vi "myRIO_BRig_RT__Case_Exp_State_Selection__v4.vi"(0 "input_dataCurrent":u16[](array[numeric]), 1 "input_state":T1, 2 "input_dataExp":u16[](array[numeric]), 5 "input_LickL":bool, 7 "input_FPGA_SelectReward":bool, 9 "input_FPGA_SelectWrong":bool, 11 "input_LickR":bool, 12 "input_arrTrig":bool[](array[boolean])) -> (3 "output_state":T1, 4 "output_dataCurrent":u16[](array[numeric]), 10 "output_LC_Event_l1":bool, 13 "output_LC_Laser_l2":bool, 14 "output_LC_Event_l2":bool, 15 "output_LC_Laser_l1":bool)   [LabVIEW 2014]
uses:
  myRIO_BRig_RT__Case_Exp_stateList.ctl
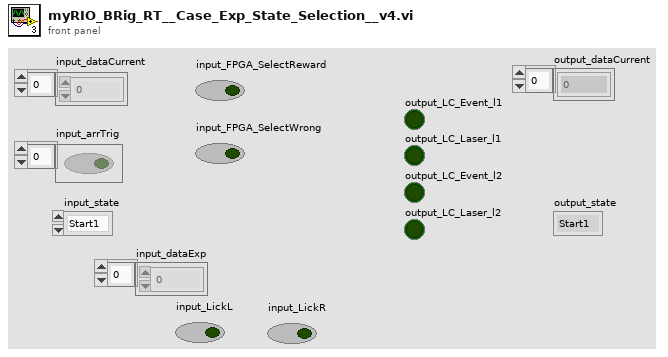
[diagram p1: front panel]
types:
  T1 = typedef "myRIO_BRig_RT__Case_Exp_stateList.ctl" = enum16{"Start1", "Start2", "Start3", "saveSettings1", "saveSettings2", "saveSettings3", "saveSettings4", "saveSettings_LC_ENL_l1", "saveSettings_LC_ENL_l2", "saveSettings_LC_Cue_l1", "saveSettings_LC_Cue_l2", "saveSettings6_LC_l1_Other", "SaveSettings6_LC_l2_Other", "setSettings_Audio", "setSettings_Laser", "initBlock_pre", "initBlock", "initBlock2", "initBlock_post", "initTrial_pre", "initTrial", "initTrial2", "initTrial3", "initTrial4", "initTrial_LC_ENL1", "initTrial_LC_Cue1", "initTrial_LC_Cue1_2", "initTrial_LC_Sel", "initTrial_post", "ENL1_pre", "ENL1", "ENL1_post", "ENL1Penalty_pre", "ENL1Penalty", "ENL2_pre", "ENL2", "ENL2Penalty_pre", "ENL2Penalty", "Cue1_pre", "Cue1", "Cue1_post", "Cue1Penalty_pre", "Cue1Penalty", "Cue2_pre", "Cue2", "Cue2Penalty_pre", "Cue2Penalty", "Selection_pre", "Selection", "Select_post", "SelectReward_pre", "SelectReward", "SelectRewardPost_pre", "SelectRewardPost", "SelectWrong_pre", "SelectWrong", "SelectWrong_post", "SelectTimeout_pre", "SelectTimeout", "SelectTimeout_post", "endTrial_pre", "endTrial1", "endTrial2", "endTrial3", "endTrial_post", "endBlock_pre", "endBlock", "endBlock_post", "endExp", "commConnect", "commUpload_pre", "commUpload_dataBlock", "commUpload_dataCurrent", "commUpload_dataExp", "commUpload_dataLC", "commUpload_dataTrial", "commUpload_post", "saveData_pre", "saveData_dataBlock", "saveData_dataCurrent", "saveData_dataExp", "saveData_dataLC", "saveData_dataTrial", "saveData_post", "empty_endBlock1", "empty_endBlock2", "empty_endTrial1", "empty_endTrial2", "empty_endTrial3", "empty_endTrial4", "empty_endTrial5", "dummyState", "dummyState_endBlock"}
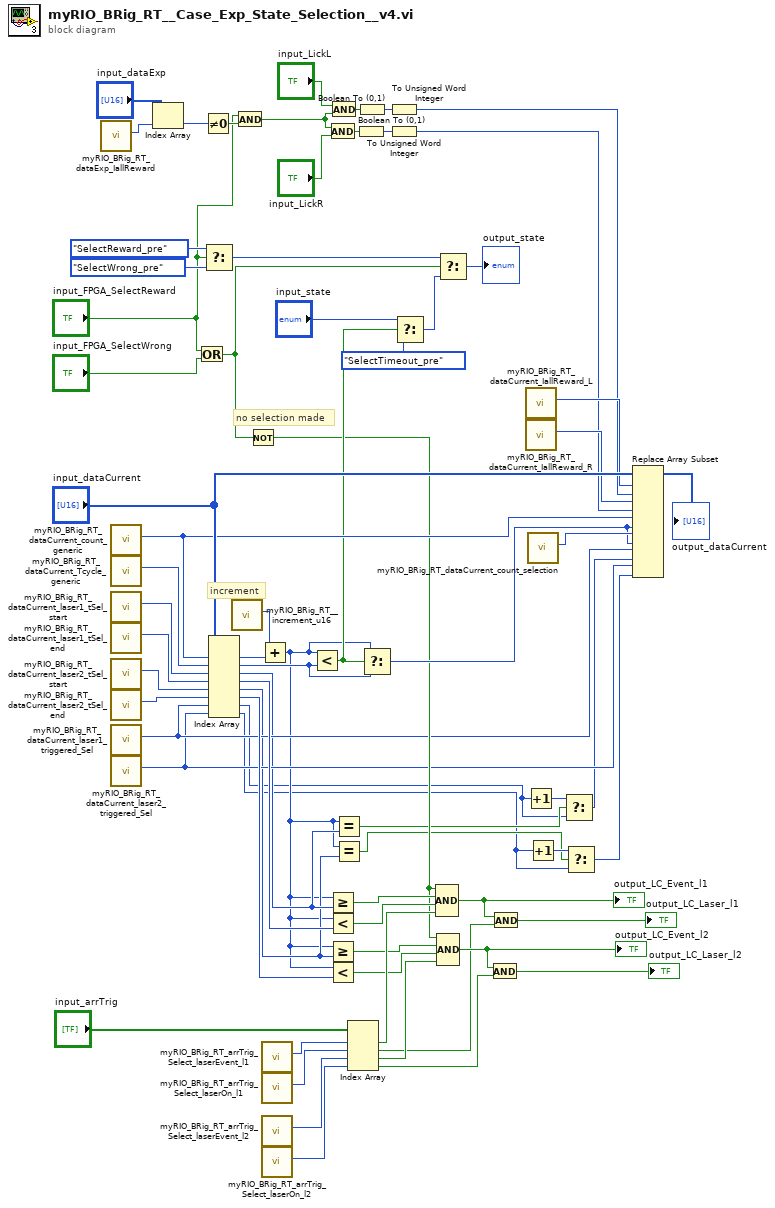
[diagram p0: block diagram]
diagram:
  # "no selection made"
  # "increment"
  n1 = call "myRIO_BRig_RT_dataExp_IallReward.vi"() -> ("output_I_allReward"=w13:i32)  [unwired: 11 in]
  n2 = call "myRIO_BRig_RT_dataCurrent_count_generic.vi"() -> ("output_count_generic"=w54:i32)  [unwired: 11 in]
  n3 = call "myRIO_BRig_RT_dataCurrent_Tcycle_generic.vi"() -> ("output_Tcycle_generic"=w66:i32)  [unwired: 11 in]
  n4 = call "myRIO_BRig_RT_dataCurrent_laser1_tSel_start.vi"() -> ("output_laser1_tSel_start"=w67:i32)  [unwired: 11 in]
  n5 = call "myRIO_BRig_RT_dataCurrent_laser1_tSel_end.vi"() -> ("output_laser1_tSel_end"=w68:i32)  [unwired: 11 in]
  n6 = call "myRIO_BRig_RT_dataCurrent_laser2_tSel_start.vi"() -> ("output_laser2_tSel_start"=w59:i32)  [unwired: 11 in]
  n7 = call "myRIO_BRig_RT_dataCurrent_laser2_tSel_end.vi"() -> ("output_laser2_tSel_end"=w58:i32)  [unwired: 11 in]
  n8 = call "myRIO_BRig_RT_dataCurrent_laser1_triggered_Sel.vi"() -> ("output_laser1_triggered_Selection"=w29:i32)  [unwired: 11 in]
  n9 = call "myRIO_BRig_RT_dataCurrent_laser2_triggered_Sel.vi"() -> ("output_laser2_triggered_Selection"=w28:i32)  [unwired: 11 in]
  n10 = Index Array(array="input_dataExp", index=w13) -> (element=w15:u16)
  n11 = Or(x="input_FPGA_SelectReward", y="input_FPGA_SelectWrong") -> (x .or. y?=w48:bool)
  n12 = Not Equal To 0?(x=w15) -> (x != 0?=w14:bool)
  n13 = Select(t=myRIO_BRig_RT__Case_Exp_stateList."SelectReward_pre" ("Enum"), s="input_FPGA_SelectReward", f=myRIO_BRig_RT__Case_Exp_stateList."SelectWrong_pre" ("Enum")) -> (s? t:f=w69:T1)
  n14 = Index Array(array="input_dataCurrent", index #1=w54, index #2=w66, index #3=w67, index #4=w68, index #5=w59, index #6=w58, index #7=w29, index #8=w28) -> (element #1=w64:u16, element #2=w52:u16, element #3=w27:u16, element #4=w57:u16, element #5=w26:u16, element #6=w56:u16, element #7=w22:u16, element #8=w19:u16)
  n15 = call "myRIO_BRig_RT__increment_u16.vi"() -> ("output_increment__u16"=w65:u16)  [unwired: 11 in]
  n16 = And(x="input_FPGA_SelectReward", y=w14) -> (x .and. y?=w5:bool)
  n17 = Not(x=w48) -> (.not. x?=w41:bool)
  n18 = Add(x=w65, y=w64) -> (x+y=w25:u16)
  n19 = call "myRIO_BRig_RT_arrTrig_Select_laserEvent_l1.vi"() -> ("output_arrTrig_Select_laserEvent_l1"=w44:i32)  [unwired: 11 in]
  n20 = call "myRIO_BRig_RT_arrTrig_Select_laserOn_l1.vi"() -> ("output_arrTrig_Select_laserOn_l1"=w43:i32)  [unwired: 11 in]
  n21 = call "myRIO_BRig_RT_arrTrig_Select_laserEvent_l2.vi"() -> ("output_arrTrig_Select_laserEvent_l2"=w31:i32)  [unwired: 11 in]
  n22 = call "myRIO_BRig_RT_arrTrig_Select_laserOn_l2.vi"() -> ("output_arrTrig_Select_laserOn_l2"=w30:i32)  [unwired: 11 in]
  n23 = Less?(x=w25, y=w52) -> (x < y?=w53:bool)
  n24 = And(x=w5, y="input_LickR") -> (x .and. y?=w8:bool)
  n25 = Greater Or Equal?(x=w25, y=w27) -> (x >= y?=w47:bool)
  n26 = Less?(x=w25, y=w57) -> (x < y?=w46:bool)
  n27 = Greater Or Equal?(x=w25, y=w26) -> (x >= y?=w40:bool)
  n28 = Less?(x=w25, y=w56) -> (x < y?=w39:bool)
  n29 = And(x="input_LickL", y=w5) -> (x .and. y?=w9:bool)
  n30 = Equal?(x=w25, y=w27) -> (x = y?=w24:bool)
  n31 = Equal?(x=w25, y=w26) -> (x = y?=w20:bool)
  n32 = Index Array(array="input_arrTrig", index #1=w44, index #2=w43, index #3=w31, index #4=w30) -> (element #1=w42:bool, element #2=w34:bool, element #3=w38:bool, element #4=w36:bool)
  n33 = Boolean To (0,1)(Boolean=w8) -> (0, 1=w6:i16)
  n34 = Boolean To (0,1)(Boolean=w9) -> (0, 1=w7:i16)
  n35 = Select(t=w25, s=w53, f=w52) -> (s? t:f=w50:u16)
  n36 = To Unsigned Word Integer(number=w7) -> (unsigned 16bit integer=w2:u16)
  n37 = To Unsigned Word Integer(number=w6) -> (unsigned 16bit integer=w1:u16)
  n38 = Select(t="input_state", s=w53, f=myRIO_BRig_RT__Case_Exp_stateList."SelectTimeout_pre" ("Enum")) -> (s? t:f=w61:T1)
  n39 = Compound Arithmetic op=AND(w41, w47, w46, w42) -> (w35:bool)
  "output_LC_Event_l1" <- w35
  n40 = Compound Arithmetic op=AND(w41, w40, w39, w38) -> (w37:bool)
  "output_LC_Event_l2" <- w37
  n41 = Select(t=w69, s=w48, f=w61) -> (s? t:f=→"output_state":T1)
  n42 = And(x=w37, y=w36) -> (x .and. y?=→"output_LC_Laser_l2":bool)
  n43 = And(x=w35, y=w34) -> (x .and. y?=→"output_LC_Laser_l1":bool)
  n44 = call "myRIO_BRig_RT_dataCurrent_IallReward_L.vi"() -> ("output_IallReward_L"=w4:i32)  [unwired: 11 in]
  n45 = call "myRIO_BRig_RT_dataCurrent_IallReward_R.vi"() -> ("output_IallReward_R"=w3:i32)  [unwired: 11 in]
  n46 = Increment(x=w22) -> (x+1=w23:u16)
  n47 = call "myRIO_BRig_RT_dataCurrent_count_selection.vi"() -> ("output_count_generic"=w51:i32)  [unwired: 11 in]
  n48 = Increment(x=w19) -> (x+1=w21:u16)
  n49 = Select(t=w23, s=w24, f=w22) -> (s? t:f=w18:u16)
  n50 = Select(t=w21, s=w20, f=w19) -> (s? t:f=w17:u16)
  n51 = Replace Array Subset(array="input_dataCurrent", new element #1=w2, index #1=w4, new element #2=w1, index #2=w3, new element #3=w50, index #3=w54, new element #4=w50, index #4=w51, new element #5=w18, index #5=w29, new element #6=w17, index #6=w28) -> (→"output_dataCurrent":u16[])
